vi "onCreateListener.vi"(6 "timeout (ms)":i32=100, 8 "error in (no error)":errorcluster, 10 "Configuration":refnum<class "WebsocketsConnection.lvclass">) -> (0 "error out":errorcluster, 3 "Listener":refnum<class "Connection.lvclass">)   [LabVIEW 2013, in "MQTT_Websockets.lvlib" / "WebsocketsConnection.lvclass"]
uses:
  WebsocketsConnection.lvclass
  MQTT_Connection/Connection/Connection.lvclass
  WebsocketsConnection.lvclass/WebsocketsConnection.ctl
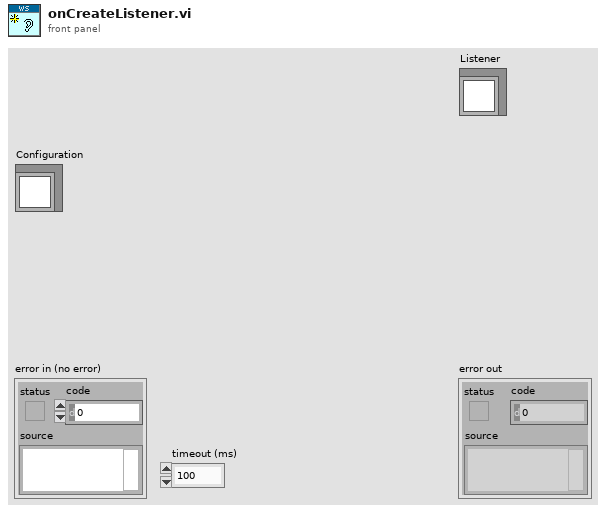
[diagram p1: front panel]
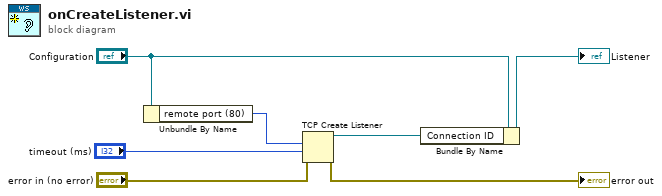
[diagram p0: block diagram]
diagram:
  n1 = Unbundle By Name("Configuration") -> ("remote port (80)"=w4:u16)
  n2 = TCP Create Listener(8:"error in (no error)", 9:"timeout (ms)", 10:w4) -> (0:→"error out":errorcluster, 3:w6:refnum<k5>)  [unwired: 2 in, 1 out]
  n3 = Bundle By Name(cluster="Configuration", "Connection ID"=w6) -> (→"Listener":refnum<class "WebsocketsConnection.lvclass">)
